vi "myRIO v1.0 AO Block Write Resource Manager.vi"(7 "Action":enum16{"Get", "Set"}(ring), 10 "AO Resource In":T1 caption="AO (N Samples) Configuration") -> (1 "Action Succeeds":bool=TRUE, 2 "AO Resource Out":T1 caption="AO (N Samples) Configuration")   [LabVIEW 2021]
uses:
  <vilib>/myRIO/Common/Instrument Driver Framework/myRIO v1.0/AO Block/typedefs/AO Block Configuration.ctl
  <vilib>/myRIO/Common/Instrument Driver Framework/myRIO v1.0/Resource Manager/vis/myRIO v1.0 Block Write Configuration.vi
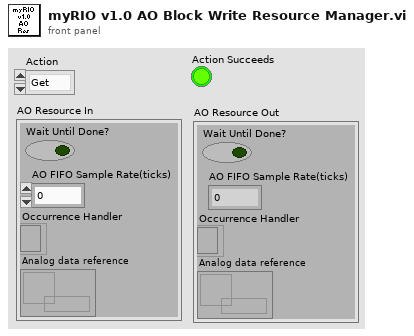
[diagram p1: front panel]
types:
  T1 = typedef "AO Block Configuration.ctl" = cluster{"Wait Until Done?":bool, "AO FIFO Sample Rate(ticks)":u32, "Occurrence Handler ":refnum<k4>, "Analog data reference":refnum<data-value>}
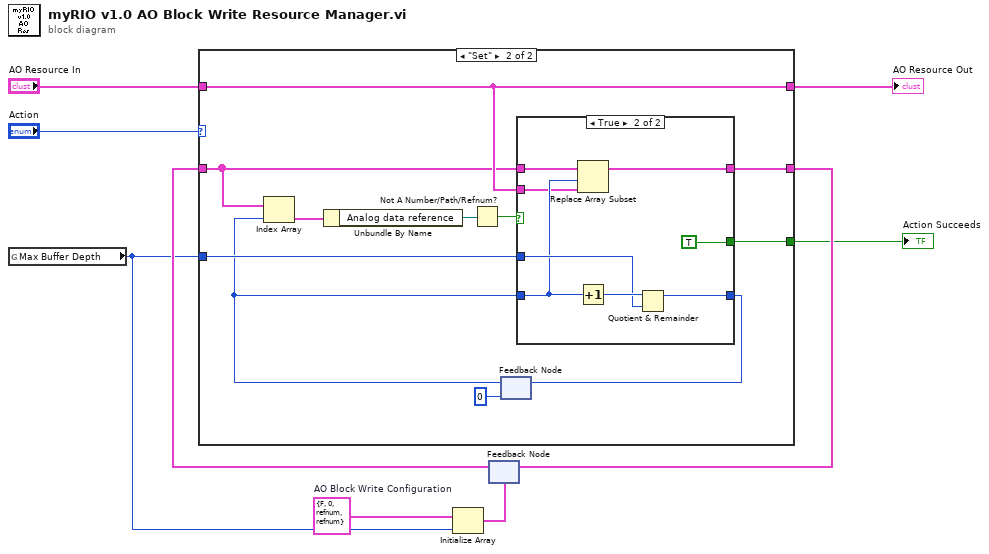
[diagram p0: block diagram]
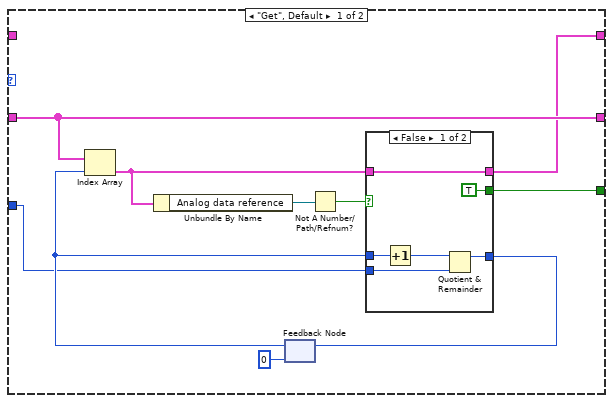
[diagram p2: hidden frame]
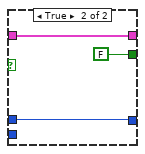
[diagram p3: hidden frame]
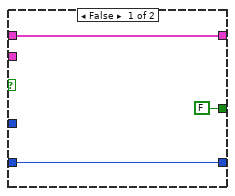
[diagram p4: hidden frame]
diagram:
  w4 = T1 {"Wait Until Done?"=FALSE, "AO FIFO Sample Rate(ticks)"=0, "Occurrence Handler "=refnum, "Analog data reference"=refnum}  # AO Block Write Configuration
  n1 = global read "myRIO v1.0 Block Write Configuration.vi" "Max Buffer Depth"() -> (w2:u32)
  n2 = Initialize Array(w4, w2) -> (w3:T1[])
  n3 = feedback #1(w3) -> (w8:T1[])
  n4 = case shown="\"Set\"" "Action" {
    tunnel: w8 -> [w19 w31]
    tunnel: [w19 w39] -> w7
    tunnel: "AO Resource In" -> [_ w37]
    tunnel: [w14 w37] -> w5
    tunnel: w2 -> [w11 w38]
    tunnel: [w13 w34] -> w1
    frame "Get", Default {
      n5 = feedback #2(u32 0) -> (w12:u32)
      n6 = Index Array(array=w19, index=w12) -> (element=w15:T1)
      n7 = Unbundle By Name(w15) -> ("Analog data reference"=w17:refnum<data-value>)
      n8 = Not A Number/Path/Refnum?(number/path/refnum=w17) -> (NaN/Path/Refnum?=w16:bool)
      n9 = case shown="False" w16 {
        tunnel: w15 -> [w24 w28]
        tunnel: [w24 w28] -> w14
        tunnel: [TRUE ("Action Succeeds") FALSE ("Action Succeeds")] -> w13
        tunnel: w12 -> [w22 w26]
        tunnel: w11 -> [w21 _]
        tunnel: [w20 w26] -> w10
        frame False {
          n10 = Increment(x=w22) -> (x+1=w23:u32)
          n11 = Quotient & Remainder(x=w23, y=w21) -> (x-y*floor(x/y)=w20:u32)  [unwired: 1 out]
        }
        frame True {
        }
      }
      n12 = feedback-in #2(w10) -> ()
    }
    frame "Set" {
      n13 = feedback #3(u32 0) -> (w30:u32)
      n14 = Index Array(array=w31, index=w30) -> (element=w29:T1)
      n15 = Unbundle By Name(w29) -> ("Analog data reference"=w36:refnum<data-value>)
      n16 = Not A Number/Path/Refnum?(number/path/refnum=w36) -> (NaN/Path/Refnum?=w35:bool)
      n17 = case shown="True" w35 {
        tunnel: w31 -> [w42 w50]
        tunnel: [w42 w49] -> w39
        tunnel: w38 -> [_ w47]
        tunnel: w30 -> [w41 w46]
        tunnel: [w41 w45] -> w32
        tunnel: w37 -> [_ w44]
        tunnel: [FALSE ("Action Succeeds") TRUE ("Action Succeeds")] -> w34
        frame False {
        }
        frame True {
          n18 = Replace Array Subset(array=w50, new element=w44, index=w46) -> (w49:T1[])
          n19 = Increment(x=w46) -> (x+1=w48:u32)
          n20 = Quotient & Remainder(x=w48, y=w47) -> (x-y*floor(x/y)=w45:u32)  [unwired: 1 out]
        }
      }
      n21 = feedback-in #3(w32) -> ()
    }
  }
  "AO Resource Out" <- w5
  "Action Succeeds" <- w1
  n22 = feedback-in #1(w7) -> ()
